vi "close.vi"(8 "error in":errorcluster, 11 "Scan Engine runtime in":refnum<class "Scan Engine runtime.lvclass">) -> (0 "error out":errorcluster)   [LabVIEW 2013, in "Scan Engine runtime.lvclass"]
doc: "Provides an interface for terminating a module instance. While this interface performs no operations, a child should close and deallocate any open references or memory."
uses:
  Scan Engine runtime.lvclass
  Scan Engine runtime.lvclass/Scan Engine runtime.ctl
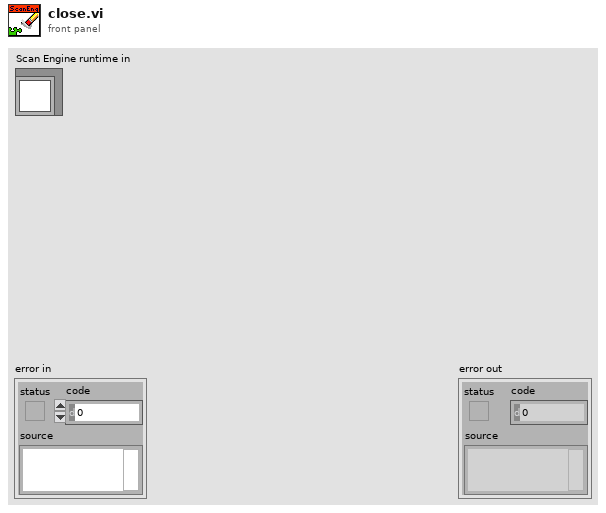
[diagram p1: front panel]
types:
  T1 = typedef "Scan Engine runtime.lvclass/Index Map.ctl" = cluster{"data type":T2, "variable ref":refnum<k21>, "index":i32}
  T2 = typedef "tag bus.lvlib/tag descriptor.lvclass/Data Type.ctl" = enum16{"Double", "Single", "I64", "I32", "I16", "I8", "U64", "U32", "U16", "U8", "Boolean", "String", "Array of Double", "Array of Single", "Array of I64", "Array of I32", "Array of I16", "Array of I8", "Array of U64", "Array of U32", "Array of U16", "Array of U8", "Array of Boolean", "Array of String"}
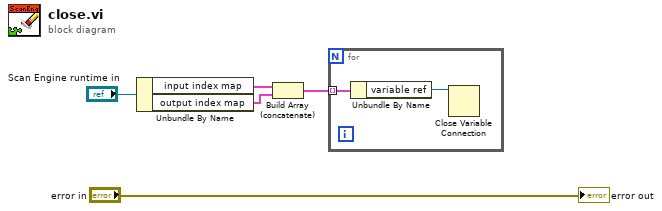
[diagram p0: block diagram]
diagram:
  n1 = Unbundle By Name("Scan Engine runtime in") -> ("input index map"=w3:T1[], "output index map"=w2:T1[])
  n2 = Build Array (concatenate)(w3, w2) -> (w1:T1[])
  n3 = for {
    tunnel: w1 -> [w7] mode=indexing
    n4 = Unbundle By Name(w7) -> ("variable ref"=w6:refnum<k21>)
    n5 = Close Variable Connection(11:w6) -> ()  [unwired: 1 in, 1 out]
  }
  "error out" <- "error in"
